vi "_Main_06_AFM.vi"() -> ()   [LabVIEW 2013]
panel:
  in  "Speed, K/min":dbl=5.0 min=0.1 max=20.0
  out "Temp, C":dbl
  out "Temp_sp, C":dbl
  out "Temp_gsp, C":dbl
  in  "Start":bool
  in  "SendPeriod, ms":dbl=20.0 min=10.0 max=10000.0
  in  "Graph every, cycle":dbl=1.0 min=1.0 max=100.0
  in  "LOG file":path=path "F:/_OneDrive/YandexDisk/YandexDisk/Компьютер MAINHOMEPC/OneDrive - Personal/_RF/_Проекты/Термоконтроллер/programming/LabView Side/Null_Log.txt"
  out "Flags":T1
  in  "Target, K":dbl=295.0 min=195.0 max=400.0
  in  "Ramp":bool
  out "Power LOG":cluster{dbl[], dbl[]}(graph)
  in  "Set temp":dbl=195.0 min=195.0 max=400.0
  in  "Setpoint":bool
  out "Vout, V":dbl format="%#.3g"
  out "Vin, V":dbl format="%#.4g"
  out "Temp, K":dbl
  out "Temp_sp, K":dbl
  out "Temp_gsp, K":dbl
  out "Temp LOG":cluster{dbl[], dbl[]}(graph)
  out "Bytes at Port":u32
  out "RecTry":i32
  in  "Stop Button":bool
  in  "COM port":refnum<visa-resource-name>
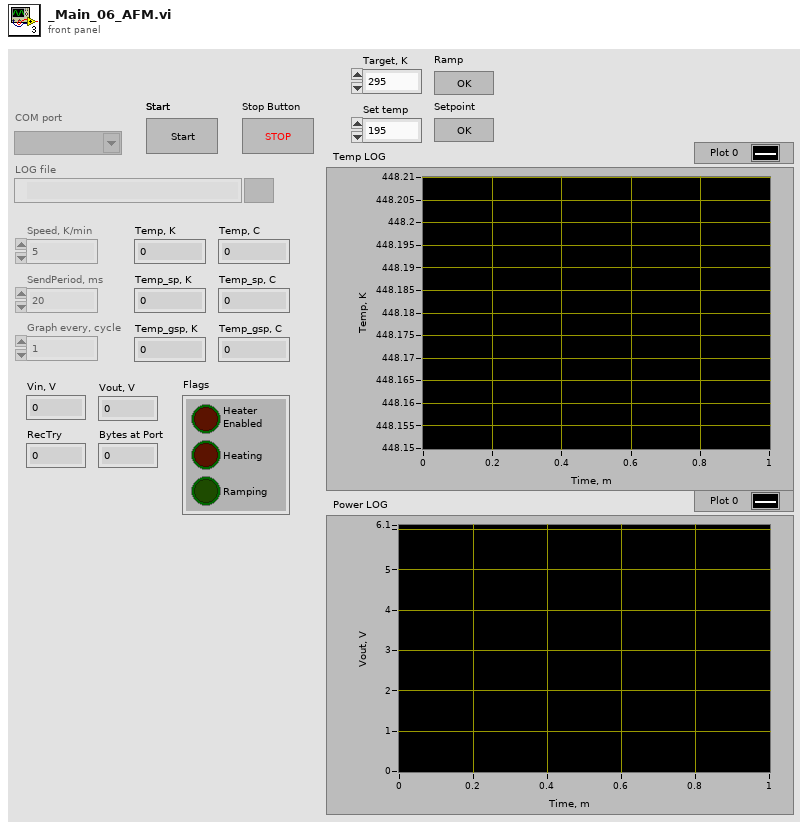
[diagram p1: front panel]
types:
  T1 = cluster{"Heater\nEnabled":bool, "Heating":bool, "Ramping":bool}
  T2 = enum8{"Enabled", "Disabled", "Disabled and Grayed Out"}
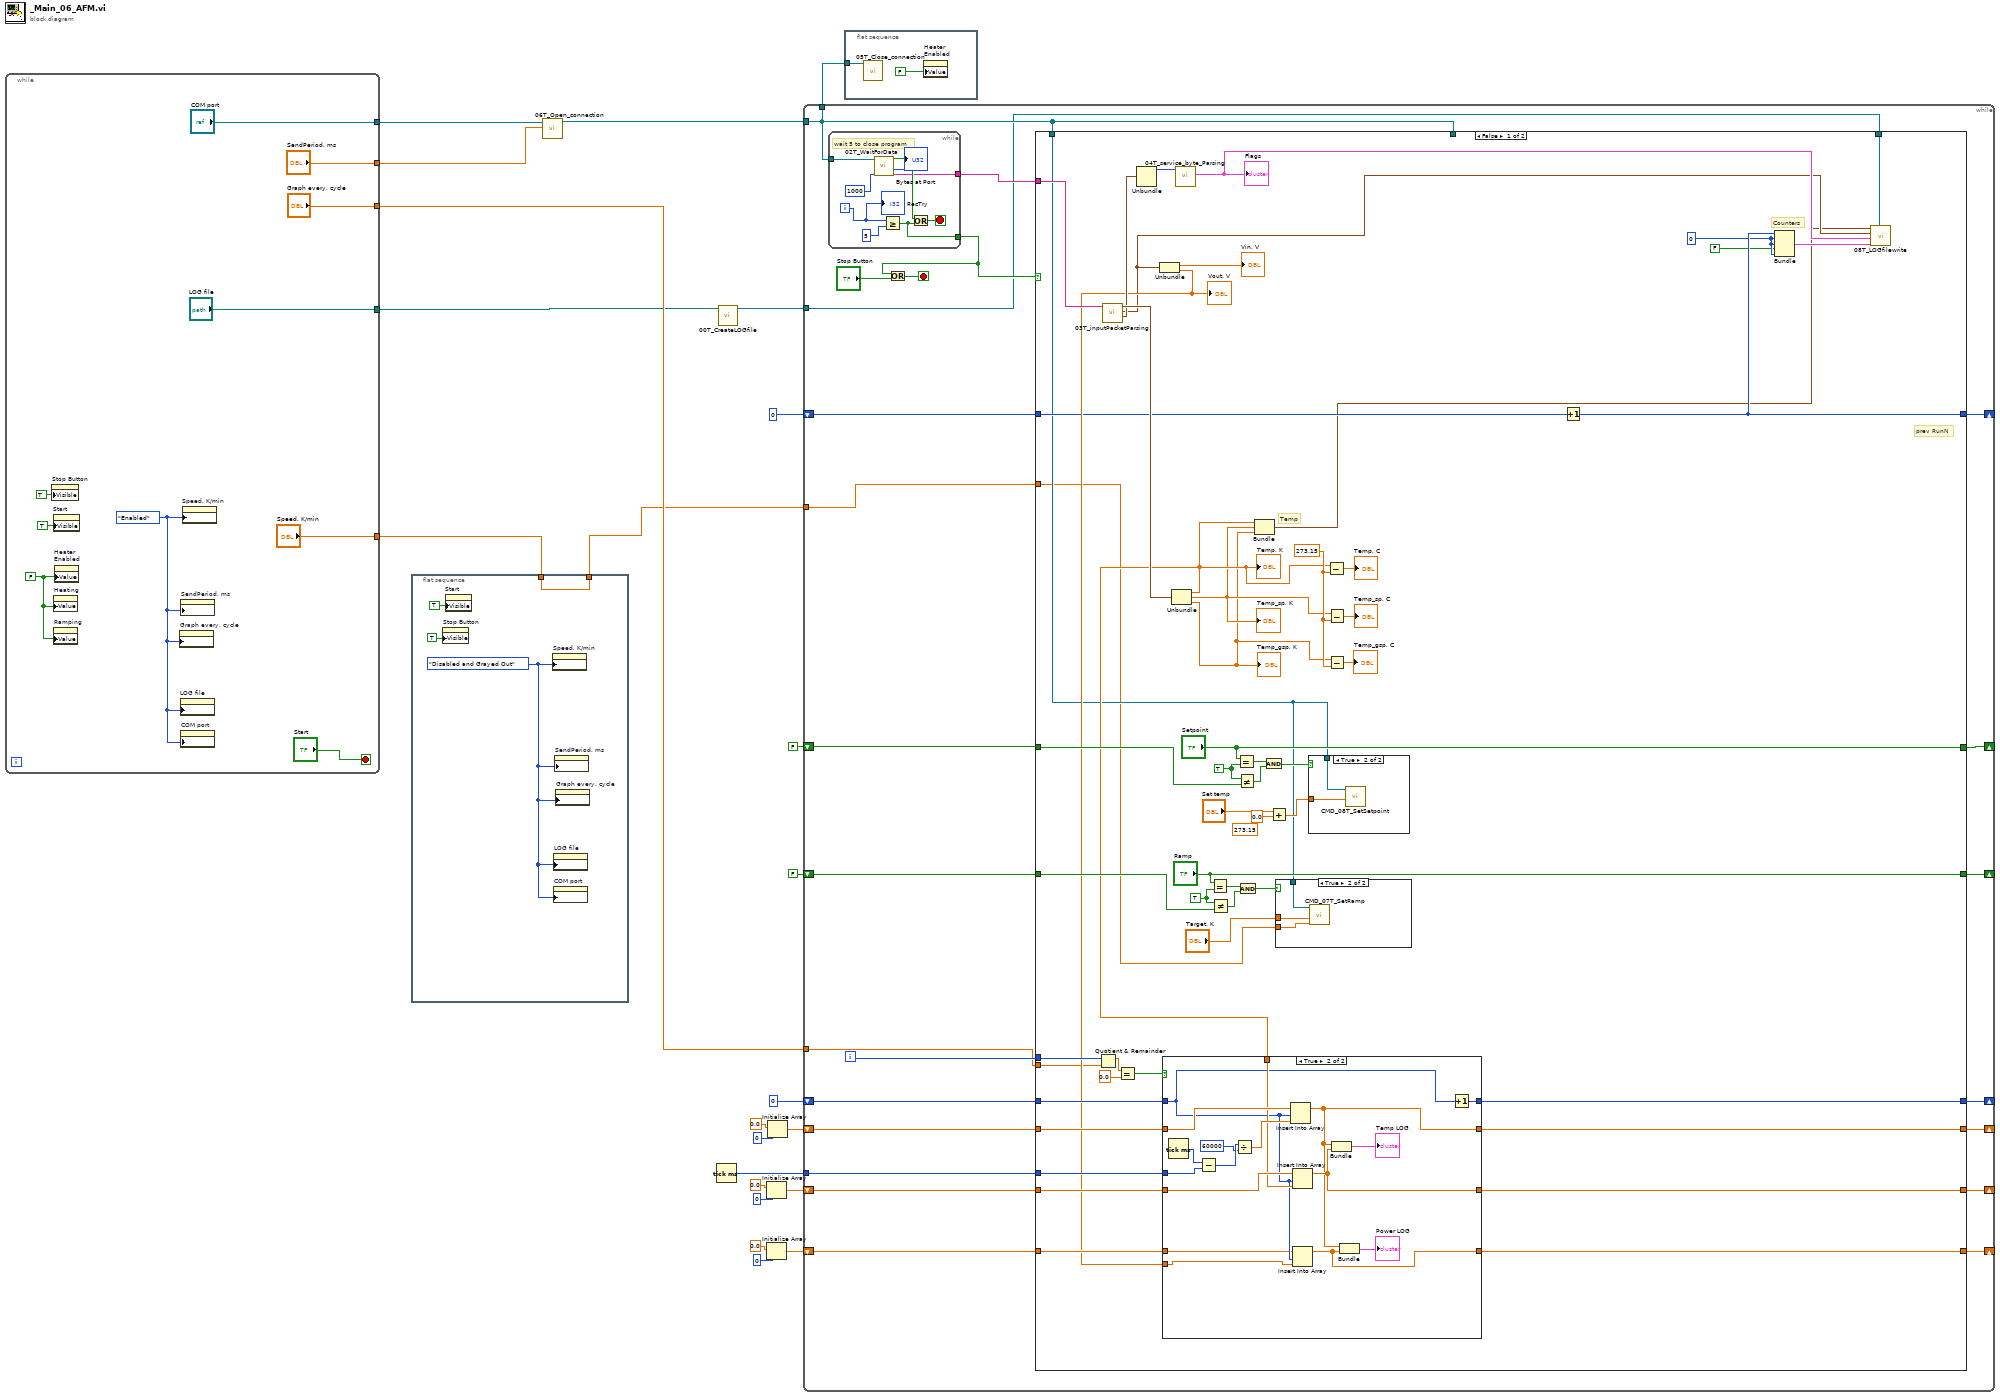
[diagram p0: block diagram]
diagram:
  n1 = while {
    tunnel: ["COM port"] -> w7
    tunnel: ["SendPeriod, ms"] -> w6
    tunnel: ["Graph every, cycle"] -> w5
    tunnel: ["LOG file"] -> w4
    tunnel: ["Speed, K/min"] -> w2
    stop <- "Start" stop-if-true
    w24 = T2."Enabled" ("Disabled")
    w25 = FALSE ("Value")
    n2 = property on="Stop Button" class="Bool"("Visible"=TRUE) -> ()  [unwired: 2 in, 2 out]
    n3 = property on="Start" class="Bool"("Visible"=TRUE) -> ()  [unwired: 2 in, 2 out]
    n4 = property on="Heating" class="Bool (strict)"("Value"=w25) -> ()  [unwired: 2 in, 2 out]
    n5 = property on="Ramping" class="Bool (strict)"("Value"=w25) -> ()  [unwired: 2 in, 2 out]
    n6 = property on="Heater\nEnabled" class="Bool (strict)"("Value"=w25) -> ()  [unwired: 2 in, 2 out]
    n7 = property on="Graph every, cycle" class="DigNum (strict)"("DisabledEnum"=w24) -> ()  [unwired: 2 in, 2 out]
    n8 = property on="LOG file" class="Path"("DisabledEnum"=w24) -> ()  [unwired: 2 in, 2 out]
    n9 = property on="SendPeriod, ms" class="DigNum (strict)"("DisabledEnum"=w24) -> ()  [unwired: 2 in, 2 out]
    n10 = property on="COM port" class="VISAName"("DisabledEnum"=w24) -> ()  [unwired: 2 in, 2 out]
    n11 = property on="Speed, K/min" class="DigNum (strict)"("DisabledEnum"=w24) -> ()  [unwired: 2 in, 2 out]
  }
  n12 = flat-sequence {
    tunnel: [w35] -> w3
    tunnel: w2 -> [w35]
    frame #0 {
      w34 = T2."Disabled and Grayed Out" ("Disabled")
      n13 = property on="Stop Button" class="Bool"("Visible"=TRUE) -> ()  [unwired: 2 in, 2 out]
      n14 = property on="Start" class="Bool"("Visible"=TRUE) -> ()  [unwired: 2 in, 2 out]
      n15 = property on="Speed, K/min" class="DigNum (strict)"("DisabledEnum"=w34) -> ()  [unwired: 2 in, 2 out]
      n16 = property on="LOG file" class="Path"("DisabledEnum"=w34) -> ()  [unwired: 2 in, 2 out]
      n17 = property on="COM port" class="VISAName"("DisabledEnum"=w34) -> ()  [unwired: 2 in, 2 out]
      n18 = property on="SendPeriod, ms" class="DigNum (strict)"("DisabledEnum"=w34) -> ()  [unwired: 2 in, 2 out]
      n19 = property on="Graph every, cycle" class="DigNum (strict)"("DisabledEnum"=w34) -> ()  [unwired: 2 in, 2 out]
    }
  }
  n20 = call "06T_Open_connection.vi"("Period, ms"=w6, "COM port"=w7) -> ("VISA"=w1:refnum<visa-resource-name>)  [unwired: 9 in]
  n21 = Tick Count (ms)() -> (millisecond timer value=w19:u32)
  n22 = call "00T_CreateLOGfile.vi"("LOG file"=w4) -> ("refnum out"=w8:refnum<file>)  [unwired: 10 in]
  n23 = Initialize Array(0.0 ("element"), 0 ("dimension size")) -> (w16:dbl[])
  n24 = Initialize Array(0.0 ("element"), 0 ("dimension size")) -> (w12:dbl[])
  n25 = Initialize Array(0.0 ("element"), 0 ("dimension size")) -> (w20:dbl[])
  n26 = while {
    tunnel: w1 -> [w47]
    tunnel: [w47] -> w10
    shift-right: [w56] -> _
    shift-left: 0 -> [w57]
    tunnel: w19 -> [w54]
    shift-right: [w52] -> _
    shift-left: w20 -> [w55]
    shift-right: [w51] -> _
    shift-left: w16 -> [w53]
    shift-right: [w49] -> _
    shift-left: FALSE ("OK Button") -> [w48]
    shift-right: [w45] -> _
    shift-left: w12 -> [w46]
    shift-right: [w44] -> _
    shift-left: FALSE ("Ramp") -> [w43]
    shift-right: [w41] -> _
    shift-left: 0 -> [w42]
    tunnel: w8 -> [w40]
    tunnel: w5 -> [w39]
    tunnel: w3 -> [w38]
    i -> [w58]
    stop <- w61 stop-if-true
    n27 = while {
      tunnel: w47 -> [w149]
      tunnel: [w152] -> w60
      tunnel: [w153] -> w59
      i -> [w151]
      stop <- w155 stop-if-true
      # "wait 5 to close program"
      n28 = call "02T_WaitForData.vi"("WaitTimeoutMS"=u32 1000, "VISA"=w149) -> ("Buffer"=w153:string, "Bytes at Port"=→"Bytes at Port":u32, "Data Recived"=w154:bool)  [unwired: 7 in]
      n29 = Greater Or Equal?(x=w151, y=5) -> (x >= y?=w152:bool)
      n30 = Or(x=w154, y=w152) -> (x .or. y?=w155:bool)
      "RecTry" <- w151
    }
    n31 = Or(x=w60, y="Stop Button") -> (x .or. y?=w61:bool)
    n32 = case shown="False" w60 {
      tunnel: w59 -> [w107 _]
      tunnel: w58 -> [w113 _]
      tunnel: w47 -> [_ _]
      tunnel: w57 -> [w111 w148]
      tunnel: [w110 w148] -> w56
      tunnel: w55 -> [w103 w147]
      tunnel: w54 -> [w109 _]
      tunnel: w53 -> [w102 w146]
      tunnel: [w108 w147] -> w52
      tunnel: [w95 w146] -> w51
      tunnel: ["Setpoint" w145] -> w49
      tunnel: w48 -> [w99 w145]
      tunnel: w47 -> [w65 _]
      tunnel: w46 -> [w91 w144]
      tunnel: [w90 w144] -> w45
      tunnel: ["Ramp" w143] -> w44
      tunnel: w43 -> [w85 w143]
      tunnel: w39 -> [w80 _]
      tunnel: w42 -> [w75 w142]
      tunnel: [w74 w142] -> w41
      tunnel: w40 -> [w66 _]
      tunnel: w38 -> [w64 _]
      frame False {
        w63 = 0
        w76 = 273.15
        w86 = TRUE ("y")
        (unwired) 273.15 ("y")
        w98 = TRUE ("x")
        # "prev RunN"
        # "Counters"
        # "Temp"
        n33 = Quotient & Remainder(x=w113, y=w80) -> (x-y*floor(x/y)=w115:dbl)  [unwired: 1 out]
        n34 = call "03T_inputPacketParsing.vi"("string"=w107) -> ("Service"=w105:cluster{i32, i32, i32, i32}, "Voltage"=w68:cluster{dbl, dbl}, "Temp"=w106:cluster{dbl, dbl, dbl})  [unwired: 7 in, 1 out]
        n35 = Equal?(x=w115, y=0.0) -> (x = y?=w112:bool)
        n36 = Unbundle(w105) -> (w82:i32)  [unwired: 3 out]
        n37 = Unbundle(w68) -> (→"Vin, V":dbl, w81:dbl)
        "Vout, V" <- w81
        n38 = Unbundle(w106) -> (w73:dbl, w72:dbl, w71:dbl)
        "Temp_gsp, K" <- w71
        "Temp_sp, K" <- w72
        "Temp, K" <- w73
        n39 = case shown="True" w112 {
          tunnel: w111 -> [w124 w130]
          tunnel: [w124 w137] -> w110
          tunnel: w103 -> [w122 w135]
          tunnel: w109 -> [_ w140]
          tunnel: w102 -> [w123 w134]
          tunnel: [w123 w132] -> w95
          tunnel: [w122 w128] -> w108
          tunnel: w73 -> [_ w131]
          tunnel: w91 -> [w121 w129]
          tunnel: [w121 w126] -> w90
          tunnel: w81 -> [_ w125]
          frame False {
          }
          frame True {
            n40 = Tick Count (ms)() -> (millisecond timer value=w141:u32)
            n41 = Subtract(x=w141, y=w140) -> (x-y=w139:u32)
            n42 = Divide(x=w139, y=u32 60000) -> (x/y=w136:dbl)
            n43 = Insert Into Array(array=w135, index=w130, new element=w136) -> (w128:dbl[])
            n44 = Insert Into Array(array=w134, index=w130, new element=w131) -> (w132:dbl[])
            n45 = Insert Into Array(array=w129, index=w130, new element=w125) -> (w126:dbl[])
            n46 = Bundle(w128, w132) -> (→"Temp LOG":cluster{dbl[], dbl[]})  [unwired: 1 in]
            n47 = Bundle(w128, w126) -> (→"Power LOG":cluster{dbl[], dbl[]})  [unwired: 1 in]
            n48 = Increment(x=w130) -> (x+1=w137:i32)
          }
        }
        n49 = call "04T_service_byte_Parsing.vi"("Service Byte"=w82) -> ("Flags"=w69:T1)  [unwired: 9 in, 1 out]
        "Flags" <- w69
        n50 = Equal?(x="Ramp", y=w86) -> (x = y?=w89:bool)
        n51 = Not Equal?(x=w86, y=w85) -> (x != y?=w88:bool)
        n52 = Equal?(x="Setpoint", y=w98) -> (x = y?=w101:bool)
        n53 = Not Equal?(x=w98, y=w99) -> (x != y?=w97:bool)
        n54 = And(x=w89, y=w88) -> (x .and. y?=w84:bool)
        n55 = Bundle(w73, w72, w71) -> (w67:cluster{dbl, dbl, dbl})  [unwired: 1 in]
        n56 = And(x=w101, y=w97) -> (x .and. y?=w96:bool)
        n57 = Add(x="Set temp", y=0.0) -> (x+y=w94:dbl)
        n58 = case shown="True" w84 {
          tunnel: w65 -> [_ w118]
          tunnel: "Target, K" -> [_ w117]
          tunnel: w64 -> [_ w116]
          frame False {
          }
          frame True {
            n59 = call "CMD_07T_SetRamp.vi"("Ramp speed, K/min"=w116, "Target, K"=w117, "VISA resource name"=w118) -> ()  [unwired: 8 in, 1 out]
          }
        }
        n60 = case shown="True" w96 {
          tunnel: w94 -> [_ w120]
          tunnel: w65 -> [_ w119]
          frame False {
          }
          frame True {
            n61 = call "CMD_08T_SetSetpoint.vi"("Setpoint, K"=w120, "VISA resource name"=w119) -> ()  [unwired: 9 in, 1 out]
          }
        }
        n62 = Subtract(x=w73, y=w76) -> (x-y=→"Temp, C":dbl)
        n63 = Subtract(x=w72, y=w76) -> (x-y=→"Temp_sp, C":dbl)
        n64 = Subtract(x=w71, y=w76) -> (x-y=→"Temp_gsp, C":dbl)
        n65 = Increment(x=w75) -> (x+1=w74:i32)
        n66 = Bundle(w74, w63, w63, "Green LED"=FALSE, w63) -> (w70:cluster{i32, i32, i32, "Green LED":bool, i32})  [unwired: 1 in]
        n67 = call "08T_LOGfilewrite.vi"("refnum out"=w66, "Counters"=w70, "Flags"=w69, "Voltage"=w68, "Temp"=w67) -> ()  [unwired: 7 in]
      }
      frame True {
      }
    }
  }
  n68 = flat-sequence {
    tunnel: w10 -> [w159]
    frame #0 {
      n69 = call "05T_Close_connection.vi"("VISA"=w159) -> ()  [unwired: 11 in]
      n70 = property on="Heater\nEnabled" class="Bool (strict)"("Value"=FALSE) -> ()  [unwired: 2 in, 2 out]
    }
  }
